vi "Tektronix DPO MSO 2000 4000 Series Acquire Multiple Digital Waveforms Example.vi"() -> ()   [LabVIEW 2010]
doc: "This example illustrates how to use autosetup and acquire multiple waveforms on multiple digital channels using the following steps:\n\n1. Specify a valid VISA session. \n2. Specify digital channels to be acquired.\n3. Specify a time-out value for reading waveform.\n4. Run the VI. The graph displays the waveforms you acquire. \n\n<B>Note:</B>\n-This VI does not work with DPO series oscilloscopes.\n- LabVIEW versions higher than 7.1 might display the data differently."
uses:
  <instrlib>/Tektronix DPO MSO 2000 4000 Series/Public/Data/Read (Multiple Digital Waveforms).vi
  <instrlib>/Tektronix DPO MSO 2000 4000 Series/Tektronix DPO MSO 2000 4000 Series.lvlib
panel:
  out "Digital Waveform Graph":digitalwaveform[](graph)
  in  "Digital Channels":u16[](array[ring])=[14] items=["Digital Channel D0"=14, "Digital Channel D1"=15, "Digital Channel D2"=16, "Digital Channel D3"=17, "Digital Channel D4"=18, "Digital Channel D5"=19, "Digital Channel D6"=20, "Digital Channel D7"=21, "Digital Channel D8"=22, "Digital Channel D9"=23, "Digital Channel D10"=24, "Digital Channel D11"=25, "Digital Channel D12"=26, "Digital Channel D13"=27, "Digital Channel D14"=28, "Digital Channel D15"=29]
  in  "Maximum Time (10000ms)":u32=10000
  in  "VISA Resource Name":refnum<visa-resource-name>
  # "(c) 2006 - 2012. National Instruments Corporation. ALL RIGHTS RESERVED."
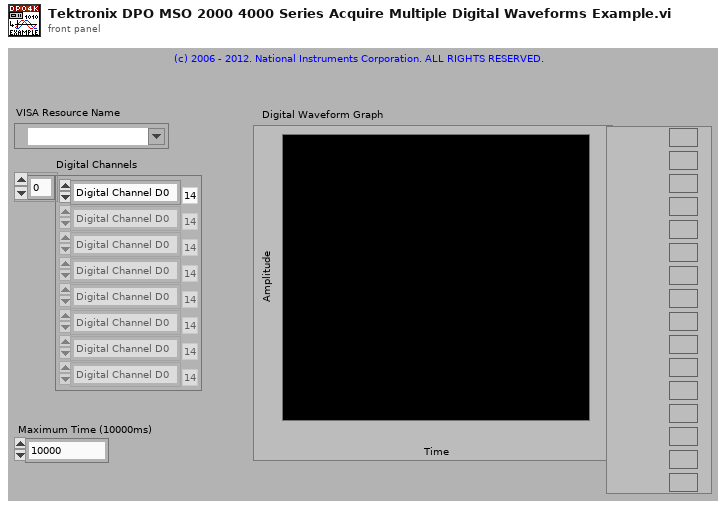
[diagram p1: front panel]
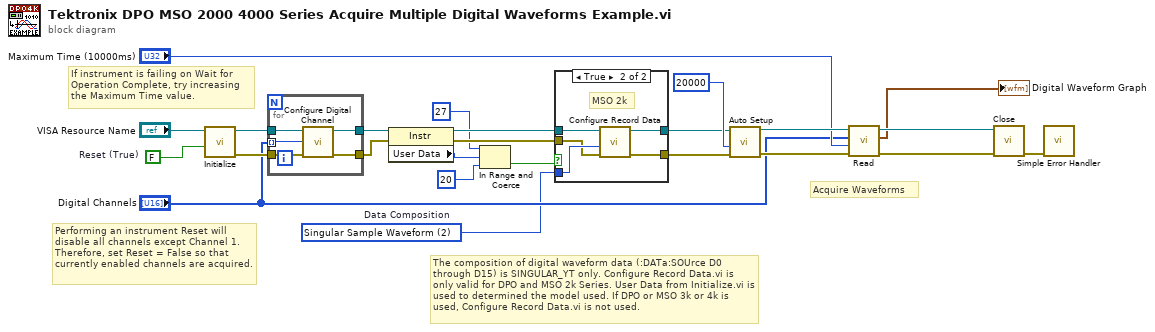
[diagram p0: block diagram]
diagram:
  w9 = u16 2 items=["Composite Sample Waveform", "Composite Peak Detect Waveform", "Singular Sample Waveform"]  # Data Composition
  w20 = FALSE  # Reset (True)
  # "The composition of digital waveform data (:DATa:SOUrce D0 through D15) is SINGULAR_YT only. Configure Record Data.vi is only valid for DPO and MSO 2k Series. User Data from Initialize.vi is used to determined the model used. If DPO or MSO 3k or 4k is used, Configure Record Data.vi is not used."
  # "Acquire Waveforms"
  # "If instrument is failing on Wait for Operation Complete, try increasing the Maximum Time value."
  # "Performing an instrument Reset will disable all channels except Channel 1. Therefore, set Reset = False so that currently enabled channels are acquired."
  n1 = call <instrlib>:"Initialize.vi"("Reset (True)"=w20, "VISA resource name"="VISA Resource Name") -> ("error out"=w18:errorcluster, "VISA resource name out"=w19:refnum<visa-resource-name>)  [unwired: 8 in]
  n2 = for {
    tunnel: w19 -> [w29]
    tunnel: w18 -> [w28]
    tunnel: [w27] -> w8
    tunnel: [w26] -> w7
    tunnel: "Digital Channels" -> [w25] mode=indexing
    n3 = call <instrlib>:"Configure Digital Channel.vi"("error in (no error)"=w28, "Digital Channel (14: Digital Channel 0)"=w25, "VISA resource name"=w29) -> ("error out"=w26:errorcluster, "VISA resource name out"=w27:refnum<visa-resource-name>)  [unwired: 7 in]
  }
  n4 = property class="Instr"(reference=w8, error in=w7) -> (reference out=w6:refnum<visa-resource-name>, error out=w5:errorcluster, "User Data"=w4:u32)
  n5 = In Range and Coerce(upper limit=u32 27, x=w4, lower limit=u32 20) -> (In Range?=w1:bool)  [unwired: 1 out]
  n6 = case shown="True" w1 {
    tunnel: [w31 w36] -> w11
    tunnel: [w30 w35] -> w10
    tunnel: w9 -> [_ w34]
    tunnel: w6 -> [w31 w33]
    tunnel: w5 -> [w30 w32]
    frame False {
      # "MSO 4k"
    }
    frame True {
      # "MSO 2k"
      n7 = call <instrlib>:"Configure Record Data.vi"("error in (no error)"=w32, "Data Composition (0: Composite Sample Waveform)"=w34, "VISA resource name"=w33) -> ("error out"=w35:errorcluster, "VISA resource name out"=w36:refnum<visa-resource-name>)  [unwired: 7 in]
    }
  }
  n8 = call <instrlib>:"Auto Setup.vi"("error in (no error)"=w10, "Maximum Time (10000ms)"=u32 20000, "VISA resource name"=w11) -> ("error out"=w15:errorcluster, "VISA resource name out"=w17:refnum<visa-resource-name>)  [unwired: 7 in]
  n9 = call-poly <instrlib>:"Read.vi"("error in (no error)"=w15, "Maximum Time (10000ms)"="Maximum Time (10000ms)", "Digital Channels"="Digital Channels", "VISA resource name"=w17) -> ("error out"=w21:errorcluster, "Digital Waveform Graph"=→"Digital Waveform Graph":digitalwaveform[], "VISA resource name out"=w22:refnum<visa-resource-name>)  [unwired: 5 in]
  n10 = call <instrlib>:"Close.vi"("error in (no error)"=w21, "VISA resource name"=w22) -> ("error out"=w23:errorcluster)  [unwired: 9 in]
  n11 = call <vilib>:"Simple Error Handler.vi"("error in (no error)"=w23) -> ()  [unwired: 4 in, 5 out]
